vi "ASM.EnqueueState.vi"(8 "error in (no error)":errorcluster, 10 "NextState":T1=enum."Init", 11 "ActorStateMachine in":refnum<class "ActorStateMachine.lvclass">) -> (0 "error out":errorcluster, 3 "ActorStateMachine out":refnum<class "ActorStateMachine.lvclass">)   [LabVIEW 2021, in "ActorStateMachine.lvlib" / "ActorStateMachine.lvclass"]
uses:
  ActorStateMachine.lvclass
  C:/Program Files (x86)/National Instruments/LabVIEW 2021/vi.lib/ActorFramework/Actor/Actor.lvclass
  _ASM.State.ctl
  <vilib>/ActorFramework/Actor/Actor.lvclass/Actor.ctl
  <vilib>/ActorFramework/Message Enqueuer/Message Enqueuer.lvclass/Message Enqueuer.ctl
  ActorStateMachine.lvclass/ActorStateMachine.ctl
  ActorStateMachine Messages/ASM.ExecuteState Msg/ASM.ExecuteState Msg.lvclass/ASM.ExecuteState Msg.ctl
  <vilib>/ActorFramework/Message Enqueuer/Init from Existing Queue.vi
  <vilib>/ActorFramework/Message Enqueuer/Enqueue.vi
  ActorStateMachine Messages/ASM.ExecuteState Msg/ASM.ExecuteState Msg.lvclass
  C:/Program Files (x86)/National Instruments/LabVIEW 2021/vi.lib/ActorFramework/Message/Message.lvclass
  <vilib>/ActorFramework/Message Priority Queue/Priority Enqueue.vi
  <vilib>/ActorFramework/Message Enqueuer/Message Enqueuer.lvclass
  <vilib>/ActorFramework/Actor/Actor.lvclass
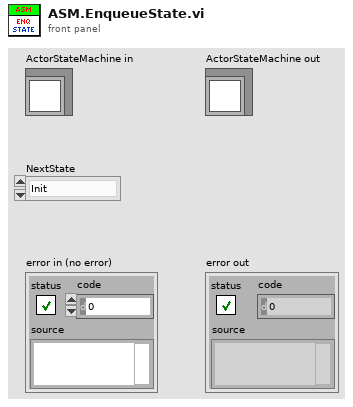
[diagram p1: front panel]
types:
  T1 = typedef "ActorStateMachine.lvlib/ActorStateMachine.lvclass/_ASM.State.ctl" = enum16{"Boom", "Pre-Init", "Init", "Post-Init", "Pre-Reset", "Reset", "Post-Reset", "Pre-Config", "Config", "Post-Config", "Pre-Ready", "Ready", "Post-Ready", "Pre-Running", "Running", "Next", "Post-Running", "Break", "Fail", "Crash", "Shutdown", "Doom"}
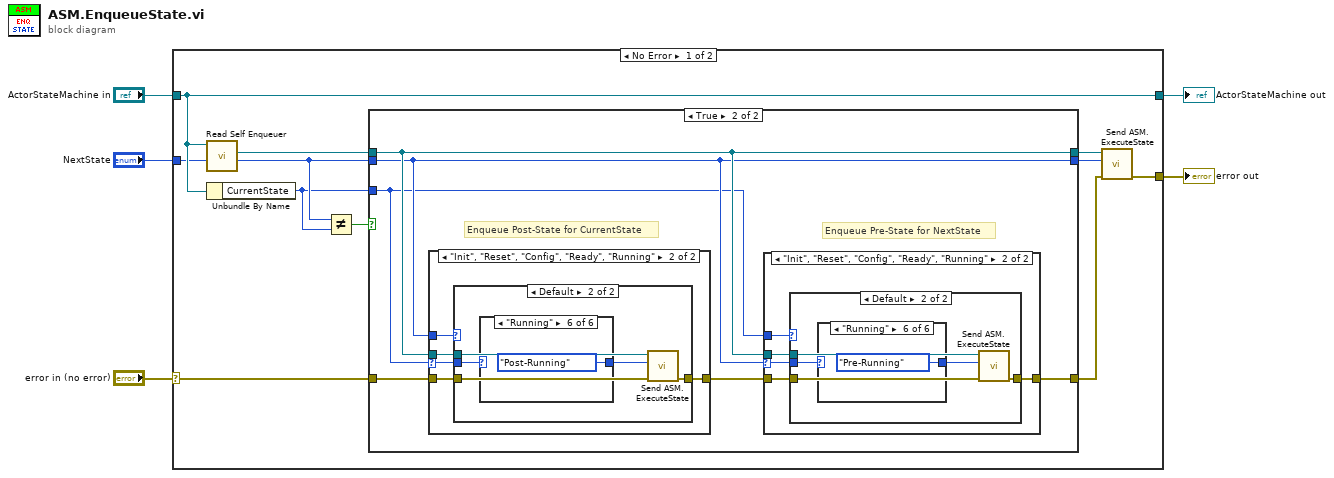
[diagram p0: block diagram]
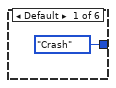
[diagram p5: hidden frame]
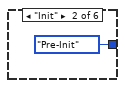
[diagram p6: hidden frame]
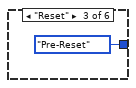
[diagram p7: hidden frame]
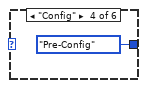
[diagram p8: hidden frame]
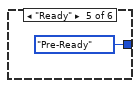
[diagram p9: hidden frame]
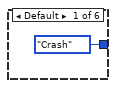
[diagram p12: hidden frame]
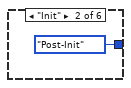
[diagram p13: hidden frame]
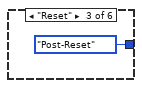
[diagram p14: hidden frame]
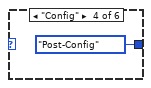
[diagram p15: hidden frame]
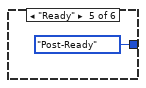
[diagram p16: hidden frame]
diagram:
  n1 = case shown="No Error" "error in (no error)" {
    selector: "error in (no error)" -> [w15 w62]
    tunnel: [w12 w62] -> w4
    tunnel: [w13 w61] -> w2
    tunnel: "ActorStateMachine in" -> [w13 w61]
    tunnel: "NextState" -> [w11 _]
    frame No Error {
      n2 = call <vilib>:"Read Self Enqueuer.vi"("Actor"=w13) -> ("Self Enqueuer"=w6:refnum<class "Message Enqueuer.lvclass">)  [unwired: 10 in]
      n3 = Unbundle By Name(w13) -> ("CurrentState"=w8:T1)
      n4 = Not Equal?(x=w11, y=w8) -> (x != y?=w10:bool)
      n5 = case shown="True" w10 {
        tunnel: w15 -> [w17 w24]
        tunnel: w6 -> [w18 w21]
        tunnel: [w17 w22] -> w14
        tunnel: w11 -> [w16 w20]
        tunnel: [w18 w21] -> w7
        tunnel: [w16 w20] -> w9
        tunnel: w8 -> [_ w19]
        frame False {
        }
        frame True {
          # "Enqueue Post-State for CurrentState"
          # "Enqueue Pre-State for NextState"
          n6 = case shown="\"Init\", \"Reset\", \"Config\", \"Ready\", \"Running\"" w19 {
            selector: w19 -> [_ w48]
            tunnel: w24 -> [w43 w46]
            tunnel: [w43 w47] -> w23
            tunnel: w21 -> [_ w45]
            tunnel: w20 -> [_ w44]
            frame Default {
            }
            frame "Init", "Reset", "Config", "Ready", "Running" {
              n7 = case shown="Default" w44 {
                tunnel: w48 -> [_ w54]
                tunnel: [w49 w53] -> w47
                tunnel: w46 -> [w49 w51]
                tunnel: w45 -> [_ w50]
                frame "Break".."Crash" {
                }
                frame Default {
                  n8 = case shown="\"Running\"" w54 {
                    tunnel: [_ASM.State."Crash" ("StateToExecute") _ASM.State."Post-Init" ("StateToExecute") _ASM.State."Post-Reset" ("StateToExecute") _ASM.State."Post-Config" ("StateToExecute") _ASM.State."Post-Ready" ("StateToExecute") _ASM.State."Post-Running" ("StateToExecute")] -> w52
                    frame Default {
                    }
                    frame "Init" {
                    }
                    frame "Reset" {
                    }
                    frame "Config" {
                    }
                    frame "Ready" {
                    }
                    frame "Running" {
                    }
                  }
                  n9 = call "Send ASM.ExecuteState.vi"("error in (no error)"=w51, "StateToExecute"=w52, "Message Enqueuer"=w50) -> ("error out"=w53:errorcluster)  [unwired: 7 in, 1 out]
                }
              }
            }
          }
          n10 = case shown="\"Init\", \"Reset\", \"Config\", \"Ready\", \"Running\"" w20 {
            selector: w20 -> [_ w30]
            tunnel: w23 -> [w25 w28]
            tunnel: [w25 w29] -> w22
            tunnel: w21 -> [_ w27]
            tunnel: w19 -> [_ w26]
            frame Default {
            }
            frame "Init", "Reset", "Config", "Ready", "Running" {
              n11 = case shown="Default" w26 {
                tunnel: w30 -> [_ w36]
                tunnel: [w31 w35] -> w29
                tunnel: w28 -> [w31 w33]
                tunnel: w27 -> [_ w32]
                frame "Break", "Crash" {
                }
                frame Default {
                  n12 = case shown="\"Running\"" w36 {
                    tunnel: [_ASM.State."Crash" ("StateToExecute") _ASM.State."Pre-Init" ("StateToExecute") _ASM.State."Pre-Reset" ("StateToExecute") _ASM.State."Pre-Config" ("StateToExecute") _ASM.State."Pre-Ready" ("StateToExecute") _ASM.State."Pre-Running" ("StateToExecute")] -> w34
                    frame Default {
                    }
                    frame "Init" {
                    }
                    frame "Reset" {
                    }
                    frame "Config" {
                    }
                    frame "Ready" {
                    }
                    frame "Running" {
                    }
                  }
                  n13 = call "Send ASM.ExecuteState.vi"("error in (no error)"=w33, "StateToExecute"=w34, "Message Enqueuer"=w32) -> ("error out"=w35:errorcluster)  [unwired: 7 in, 1 out]
                }
              }
            }
          }
        }
      }
      n14 = call "Send ASM.ExecuteState.vi"("error in (no error)"=w14, "StateToExecute"=w9, "Message Enqueuer"=w7) -> ("error out"=w12:errorcluster)  [unwired: 7 in, 1 out]
    }
    frame Error {
    }
  }
  "error out" <- w4
  "ActorStateMachine out" <- w2
